vi "DriveExecute.vi"(8 "error in (no error)":errorcluster) -> (0 "error out":errorcluster)   [LabVIEW 2020]
doc: "Execute for Drie\n\nClosed control loop for drive\n\ninput: \n error in (cluster)\n\noutput:\n error out (cluster)"
uses:
  <vilib>/Rock Robotics/WPI/ThirdParty/JAS_Junk/TrajLib/TypeDef/SWERVE_DRIVE_MODULE_STATE.ctl
  <vilib>/Rock Robotics/WPI/ThirdParty/JAS_Junk/TrajLib/TypeDef/ROTATION2D.ctl
  <vilib>/Rock Robotics/WPI/ThirdParty/JAS_Junk/TrajLib/LinearFilter_ResetToValue.vi
  <vilib>/Rock Robotics/WPI/ThirdParty/JAS_Junk/TrajLib/LinearFilter_Calculate.vi
  DriveGlobal.vi
  <vilib>/Rock Robotics/WPI/ThirdParty/JAS_Junk/TrajLib/LinearFilter_MovingAverage.vi
  <vilib>/Rock Robotics/WPI/ThirdParty/JAS_Junk/TrajLib/LinearFilter_LowPassBW1.vi
  <vilib>/Rock Robotics/WPI/ThirdParty/JAS_Junk/TrajLib/LinearFilter_LowPassBW2.vi
  <vilib>/Rock Robotics/WPI/ThirdParty/JAS_Junk/TrajLib/LinearFilter_HighPassBW1.vi
  <vilib>/Rock Robotics/WPI/ThirdParty/JAS_Junk/TrajLib/LinearFilter_HighPassBW2.vi
  <vilib>/Rock Robotics/WPI/ThirdParty/JAS_Junk/TrajLib/Trajectory_Library.lvlib
panel:
  out "ModuleStates":T1[](array[typedef]) {"Angle"."SIN" format="%13.4f"; "Angle"."COS" format="%13.4f"; "Angle"."VALUE" format="%13.4f"}
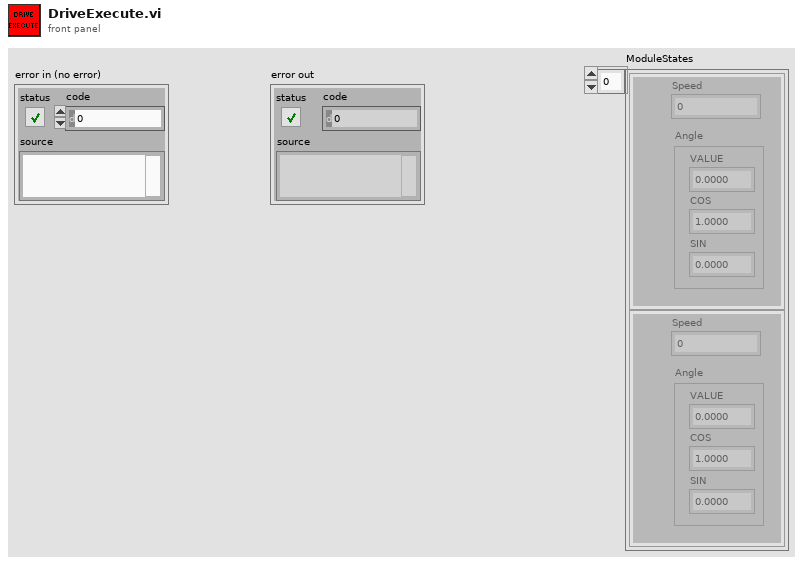
[diagram p1: front panel]
types:
  T1 = typedef "Trajectory_Library.lvlib/SWERVE_DRIVE_MODULE_STATE.ctl" = cluster{"Speed":dbl, "Angle":T2}
  T2 = typedef "Trajectory_Library.lvlib/ROTATION2D.ctl" = cluster{"VALUE":dbl, "COS":dbl, "SIN":dbl}
  T3 = enum16{"Moving Average", "Low Pass 1st Order Butterworth", "Low Pass 2nd Order Butterworth", "High Pass 1st Order Butterworth", "High Pass 2nd Order Butterworth"}
  T4 = typedef "ADIS16470 Device Reference.ctl" = cluster{"DevStatus":errorcluster, "Hardware Config":T5, "Calibration Complete":refnum<notifier>, "Status Reference":refnum<data-value>, "Data Reference":refnum<data-value>, "Sychronous Process VI":T9, "Cmd FIFO":refnum<k33>, "Source":T10, "Data FIFO":refnum<k33>, "Calibration Time (ms)":u32, "Data Reference":refnum<data-value>}
  T5 = typedef "ADIS16470 Hardware Configuration.ctl" = cluster{"SPI Clock Rate (Hz)":dbl, "IMU SPI Mode (3)":T6, "IMU Reset Pin":T7, "IMU SPI Bus":T8, "IMU Data Ready Pin":T7, "Stall Config":cluster{"Pow2BytesPerRead":u8, "StallTicks":u16, "CsToSclkTicks":u8}}
  T6 = typedef "WPI_SPIMode.ctl" = enum16{"Mode 0 (Clk Idle Low,Sample on Leading)", "Mode 1 (Clk Idle Low,Sample on Trailing)", "Mode 2 (Clk Idle High,Sample on Leading)", "Mode 3 (Clk Idle High,Sample on Trailing)"}
  T7 = typedef "FPGA_DIOChannel.ctl" = enum8{"DIO 0", "DIO 1", "DIO 2", "DIO 3", "DIO 4", "DIO 5", "DIO 6", "DIO 7", "DIO 8", "DIO 9", "DIO MXP 0", "DIO MXP 1", "DIO MXP 2", "DIO MXP 3", "DIO MXP 4", "DIO MXP 5", "DIO MXP 6", "DIO MXP 7", "DIO MXP 8", "DIO MXP 9", "DIO MXP 10", "DIO MXP 11", "DIO MXP 12", "DIO MXP 13", "DIO MXP 14", "DIO MXP 15", "SPI Port CS1", "SPI Port CS2", "SPI Port CS3", "SPI Port MISO", "SPI Port MOSI", "Invalid"}
  T8 = typedef "spi_bus.ctl" = enum16{"SPI On-Board, CS0", "SPI On-Board, CS1", "SPI On-Board, CS2", "SPI On-Board, CS3", "SPI MXP", "Invalid"}
  T9 = typedef "ADIS16470 Process.ctl" = refnum<vi>
  T10 = typedef "FPGA_CounterEncoderSourceConvertionLVSourceType.ctl" = cluster{"DevStatus":errorcluster, "AnalogTriggerMode?":bool, "DigitalMode":cluster{"DIO Channel":T11}, "AnalogTriggerMode":cluster{"AnalogTriggerIndex":T12, "OutputType":T13}}
  T11 = typedef "FPGA_DIODigitalSourceChannel.ctl" = enum8{"DIO 0", "DIO 1", "DIO 2", "DIO 3", "DIO 4", "DIO 5", "DIO 6", "DIO 7", "DIO 8", "DIO 9", "DIO MXP 0", "DIO MXP 1", "DIO MXP 2", "DIO MXP 3", "DIO MXP 4", "DIO MXP 5", "DIO MXP 6", "DIO MXP 7", "DIO MXP 8", "DIO MXP 9", "DIO MXP 10", "DIO MXP 11", "DIO MXP 12", "DIO MXP 13", "DIO MXP 14", "DIO MXP 15", "SPI Port CS1", "SPI Port CS2", "SPI Port CS3", "SPI Port MISO", "SPI Port MOSI", "Disabled"}
  T12 = typedef "FPGA_AnalogTriggerIndex.ctl" = enum8{"Trig 0", "Trig 1", "Trig 2", "Trig 3", "Trig 4", "Trig 5", "Trig 6", "Trig 7", "Invalid"}
  T13 = typedef "FPGA_AnalogTriggerOutType.ctl" = enum16{"InWindow", "TriggerState", "Rising", "Falling"}
  T14 = typedef "ADIS16470 Status.ctl" = cluster{"Calibrated?":bool, "IMU Detected?":bool}
  T15 = typedef "ADIS16470 Data.ctl" = cluster{"XAngle":dbl, "YAngle":dbl, "ZAngle":dbl}
  T16 = typedef "Trajectory_Library.lvlib/SWERVE_DRIVE_KINEMATICS.ctl" = cluster{"NumModules":i32, "InverseKinematics":T17, "ForwardKinematics":T17, "Modules":T18[], "PrevCoR":T18, "SavedModuleStates":T1[]}
  T17 = typedef "NI_Matrix.lvlib/RealMatrix.ctl" = dbl[][]
  T18 = typedef "Trajectory_Library.lvlib/TRANSLATION2D.ctl" = cluster{"X":dbl, "Y":dbl}
  T19 = typedef "Trajectory_Library.lvlib/CHASSIS_SPEEDS.ctl" = cluster{"vX":dbl, "vY":dbl, "vOmega":dbl}
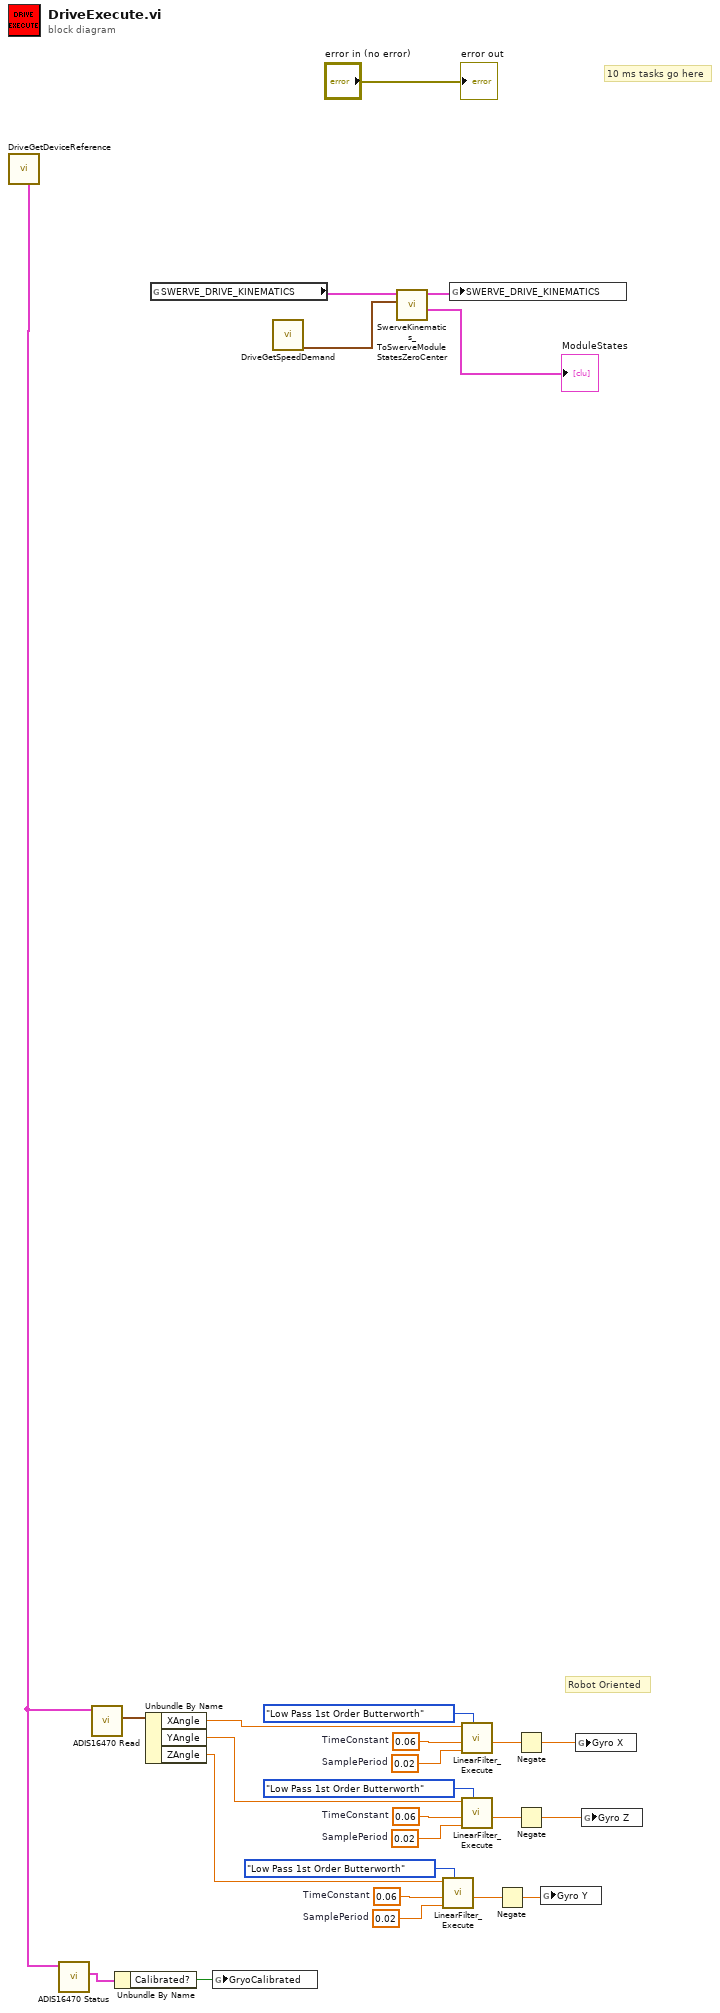
[diagram p0: block diagram]
diagram:
  w10 = 0.02  # SamplePeriod
  w9 = 0.06  # TimeConstant
  w16 = 0.02  # SamplePeriod
  w15 = 0.06  # TimeConstant
  w21 = 0.02  # SamplePeriod
  w20 = 0.06  # TimeConstant
  # "Robot Oriented"
  # "10 ms tasks go here"
  n1 = call "DriveGetDeviceReference.vi"() -> ("Gryo"=w22:T4)  [unwired: 7 in, 4 out]
  n2 = call <vilib>:"ADIS16470 Status.vi"("ADIS16470DevRef"=w22) -> ("ADIS16470 Status"=w24:T14)  [unwired: 8 in, 2 out]
  n3 = call <vilib>:"ADIS16470 Read.vi"("ADIS16470DevRef"=w22) -> ("ADIS16470 Value"=w26:T15)  [unwired: 7 in, 3 out]
  n4 = Unbundle By Name(w24) -> ("Calibrated?"=w23:bool)
  n5 = Unbundle By Name(w26) -> ("XAngle"=w5:dbl, "YAngle"=w12:dbl, "ZAngle"=w18:dbl)
  n6 = global read "DriveGlobal.vi" "SWERVE_DRIVE_KINEMATICS"() -> (w4:T16)
  n7 = global write "DriveGlobal.vi" "GryoCalibrated"(w23) -> ()
  n8 = call "DriveGetSpeedDemand.vi"() -> ("ChassisSpeedDemand"=w3:T19)  [unwired: 8 in, 3 out]
  n9 = call <vilib>:"SwerveKinematics_ToSwerveModuleStatesZeroCenter.vi"("ChassisSpeeds"=w3, "in SWERVE_DRIVE_KINEMATICS"=w4) -> ("ModuleStates"=→"ModuleStates":T1[], "out SWERVE_DRIVE_KINEMATICS"=w2:T16)  [unwired: 8 in]
  n10 = call <vilib>:"LinearFilter_Execute.vi"("Filter Type"=T3."Low Pass 1st Order Butterworth", "SamplePeriod"=w21, "TimeConstant"=w20, "Input"=w18) -> ("Output"=w17:dbl)  [unwired: 6 in, 1 out]
  n11 = global write "DriveGlobal.vi" "SWERVE_DRIVE_KINEMATICS"(w2) -> ()
  n12 = call <vilib>:"LinearFilter_Execute.vi"("Filter Type"=T3."Low Pass 1st Order Butterworth", "SamplePeriod"=w10, "TimeConstant"=w9, "Input"=w5) -> ("Output"=w7:dbl)  [unwired: 6 in, 1 out]
  n13 = call <vilib>:"LinearFilter_Execute.vi"("Filter Type"=T3."Low Pass 1st Order Butterworth", "SamplePeriod"=w16, "TimeConstant"=w15, "Input"=w12) -> ("Output"=w13:dbl)  [unwired: 6 in, 1 out]
  n14 = Negate(x=w17) -> (-x=w25:dbl)
  n15 = Negate(x=w7) -> (-x=w6:dbl)
  n16 = Negate(x=w13) -> (-x=w11:dbl)
  n17 = global write "DriveGlobal.vi" "Gyro Y"(w25) -> ()
  n18 = global write "DriveGlobal.vi" "Gyro X"(w6) -> ()
  n19 = global write "DriveGlobal.vi" "Gyro Z"(w11) -> ()
  "error out" <- "error in (no error)"
